vi "updateWarning.vi"(10 "className":string, 11 "folder":path) -> (2 "warningText":string, 3 "ok?":bool)   [LabVIEW 2023]
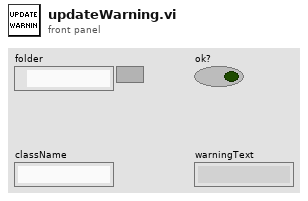
[diagram p1: front panel]
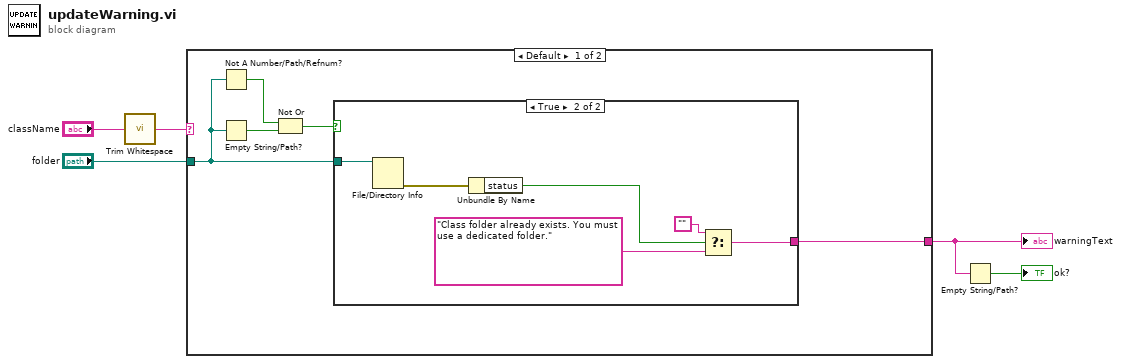
[diagram p0: block diagram]
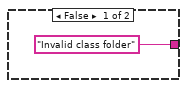
[diagram p2: hidden frame]
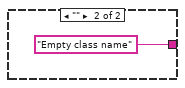
[diagram p3: hidden frame]
diagram:
  n1 = call <vilib>:"Trim Whitespace.vi"("string"="className") -> ("trimmed string"=w4:string)  [unwired: 1 in]
  n2 = case shown="Default" w4 {
    tunnel: [w7 "Empty class name" ("warningText")] -> w2
    tunnel: "folder" -> [w6 _]
    frame Default {
      n3 = Not A Number/Path/Refnum?(number/path/refnum=w6) -> (NaN/Path/Refnum?=w10:bool)
      n4 = Empty String/Path?(string/path=w6) -> (empty?=w9:bool)
      n5 = Not Or(1:w9, 2:w10) -> (0:w8:bool)
      n6 = case shown="True" w8 {
        tunnel: ["Invalid class folder" ("warningText") w12] -> w7
        tunnel: w6 -> [_ w17]
        frame False {
        }
        frame True {
          n7 = File/Directory Info(path=w17) -> (error out=w16:errorcluster)  [unwired: 1 in, 6 out]
          n8 = Unbundle By Name(w16) -> ("status"=w15:bool)
          n9 = Select(t="", s=w15, f="Class folder already exists. You must use a dedicated folder." ("warningText")) -> (s? t:f=w12:string)
        }
      }
    }
    frame "" {
    }
  }
  "warningText" <- w2
  n10 = Empty String/Path?(string/path=w2) -> (empty?=→"ok?":bool)
